vi "Insert Object in Map.vi"(0 "Robot":cluster{"Col":dbl, "Row":dbl, "Bearing":dbl}, 1 "Map":i8[][](array[numeric])=array301x301[90601 elements], 2 "Objects bottom cords":T1(array[cluster]), 3 "Grid size (m)":dbl=0.1, 5 "# safety grids":i32=4) -> (6 "Updated Map":i8[][](array[numeric]), 7 "Points":cluster{"Col":i8, "Row":i8}[](array[cluster]))   [LabVIEW 2009]
panel:
  in  "Point":cluster{"Col":i8, "Row":i8}
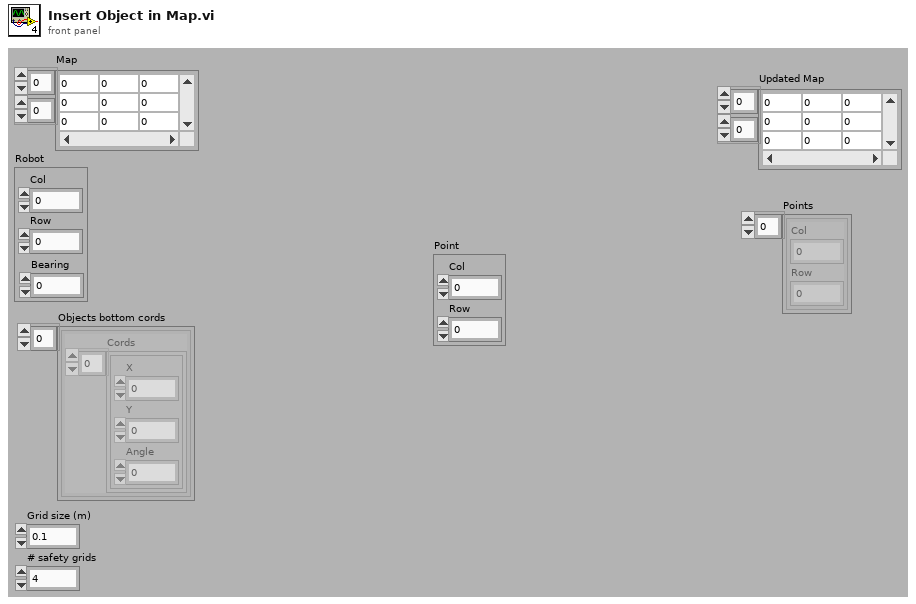
[diagram p1: front panel]
types:
  T1 = cluster{"Cords":cluster{"X":dbl, "Y":dbl, "Angle":dbl}[]}[]
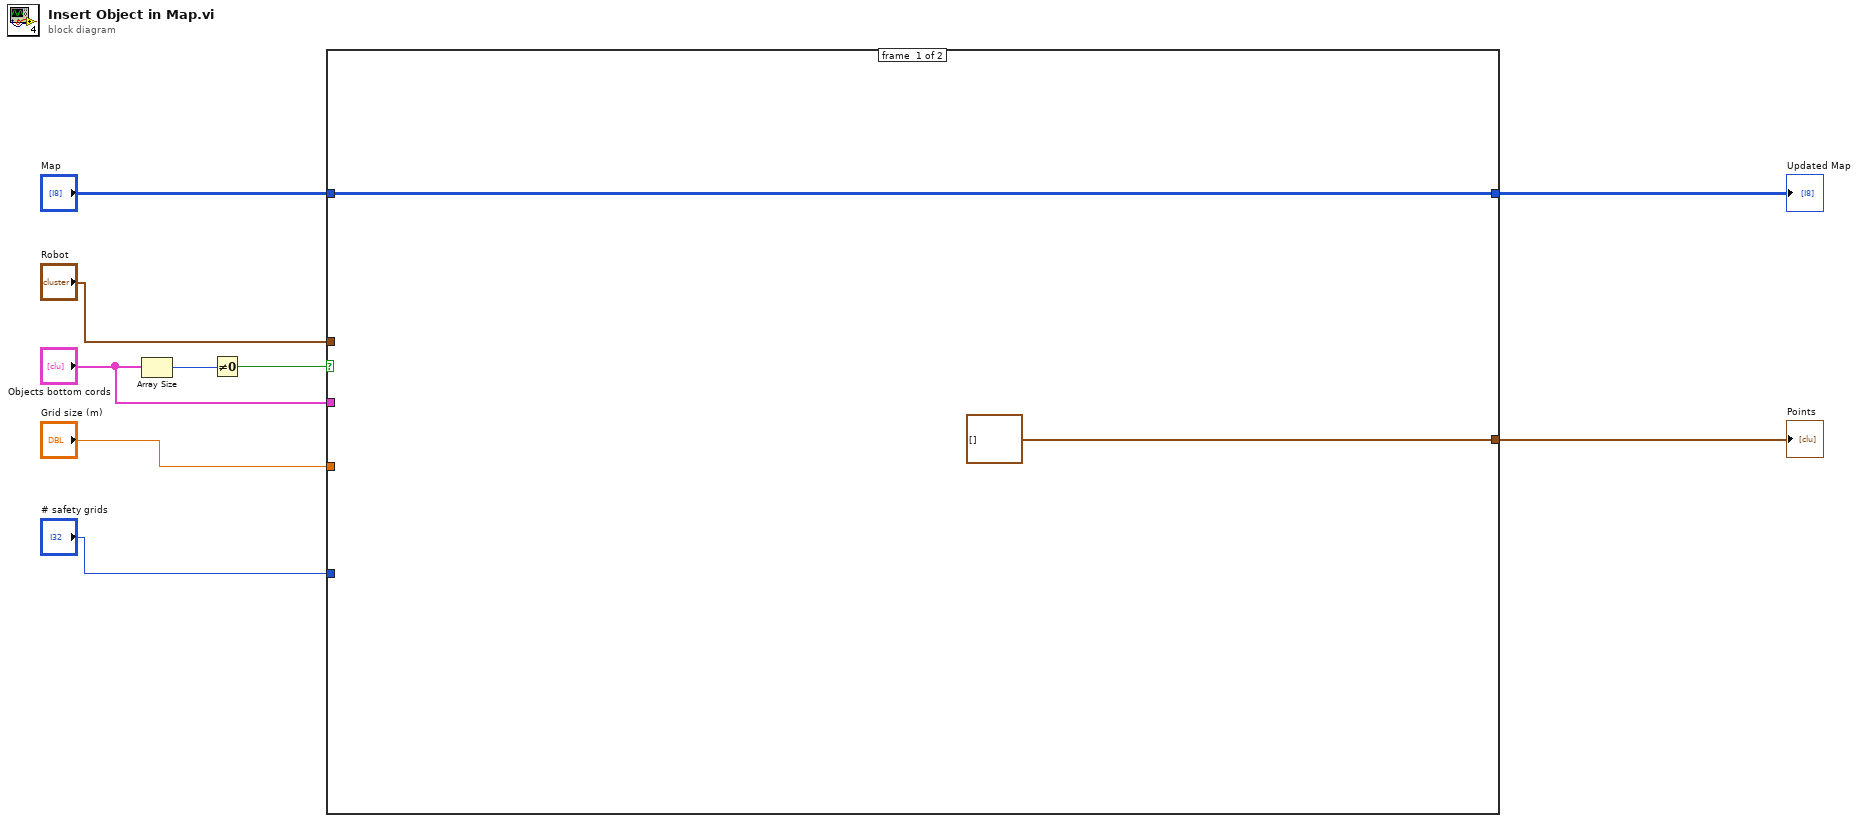
[diagram p0: block diagram]
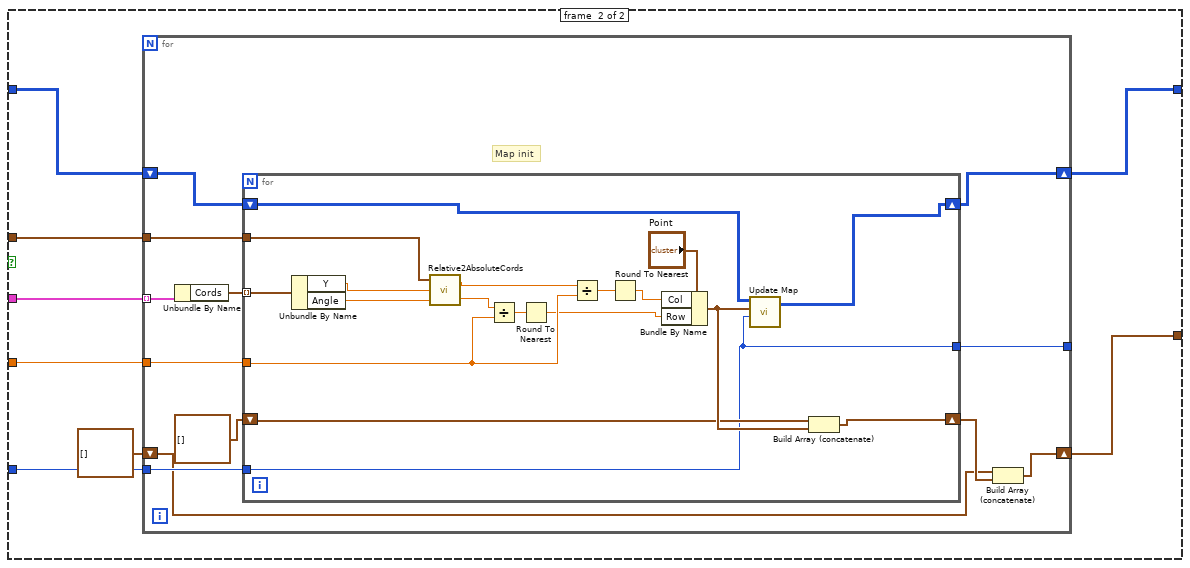
[diagram p2: hidden frame]
diagram:
  n1 = Array Size(array="Objects bottom cords") -> (size(s)=w9:i32)
  n2 = Not Equal To 0?(x=w9) -> (x != 0?=w8:bool)
  n3 = case shown="True" w8 {
    tunnel: [w11 w12] -> w6
    tunnel: "Map" -> [w11 w14]
    tunnel: [cluster{"Col":dbl, "Row":dbl}[] [] ("Points") w13] -> w5
    tunnel: "Robot" -> [_ w19]
    tunnel: "Grid size (m)" -> [_ w18]
    tunnel: "# safety grids" -> [_ w17]
    tunnel: "Objects bottom cords" -> [_ w15]
    frame #0 {
    }
    frame #1 {
      n4 = for {
        tunnel: w15 -> [w31] mode=indexing
        tunnel: w18 -> [w29]
        tunnel: w17 -> [w28]
        tunnel: [w27] -> _
        shift-right: [w24] -> w13
        shift-left: cluster{"Col":dbl, "Row":dbl}[] [] -> [w23]
        tunnel: w19 -> [w22]
        shift-right: [w21] -> w12
        shift-left: w14 -> [w20]
        # "Map init"
        n5 = Unbundle By Name(w31) -> ("Cords"=w30:cluster{"X":dbl, "Y":dbl, "Angle":dbl}[])
        n6 = for {
          tunnel: w30 -> [w49] mode=indexing
          tunnel: w29 -> [w45]
          tunnel: w28 -> [w37]
          tunnel: [w37] -> w27
          shift-right: [w39] -> w25
          shift-left: cluster{"Col":dbl, "Row":dbl}[] [] -> [w38]
          tunnel: w22 -> [w36]
          shift-right: [w35] -> w21
          shift-left: w20 -> [w34]
          n7 = Unbundle By Name(w49) -> ("Y"=w48:dbl, "Angle"=w47:dbl)
          n8 = call "Relative2AbsoluteCords.vi"("Obj bearing"=w47, "Obj distance"=w48, "Robot"=w36) -> ("Obj Y-cord"=w46:dbl, "Obj X-cord"=w44:dbl)
          n9 = Divide(x=w46, y=w45) -> (x/y=w42:dbl)
          n10 = Round To Nearest(number=w42) -> (nearest integer value=w32:dbl)
          n11 = Divide(x=w44, y=w45) -> (x/y=w43:dbl)
          n12 = Round To Nearest(number=w43) -> (nearest integer value=w33:dbl)
          n13 = Bundle By Name(cluster="Point", "Col"=w33, "Row"=w32) -> (w40:cluster{"Col":i8, "Row":i8})
          n14 = call "Update Map.vi"("# safety grids"=w37, "Point"=w40, "Map"=w34) -> ("Updated Map"=w35:i8[][])  [unwired: 2 in]
          n15 = Build Array (concatenate)(w38, w40) -> (w39:cluster{"Col":dbl, "Row":dbl}[])
        }
        n16 = Build Array (concatenate)(w23, w25) -> (w24:cluster{"Col":dbl, "Row":dbl}[])
      }
    }
  }
  "Points" <- w5
  "Updated Map" <- w6
